vi "read_ini_file.vi"() -> ()   [LabVIEW 2021]
uses:
  <vilib>/Utility/config.llb/Read Key (String).vi
  <vilib>/Utility/config.llb/NI_LVConfig.lvlib
panel:
  out "values":string[][](array[string])
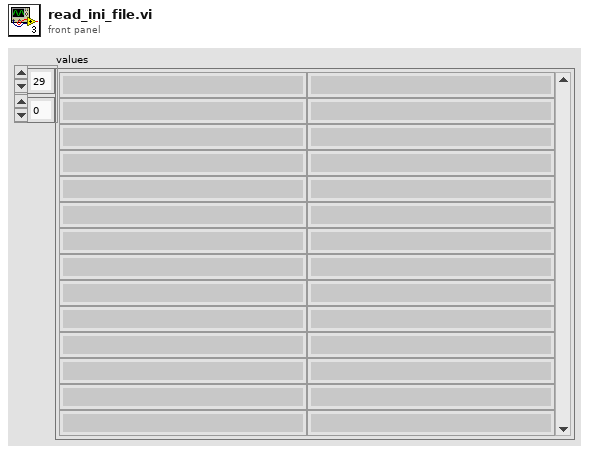
[diagram p1: front panel]
types:
  T1 = typedef "NI_LVConfig.lvlib/Config Data RefNum.ctl" = refnum<k1>
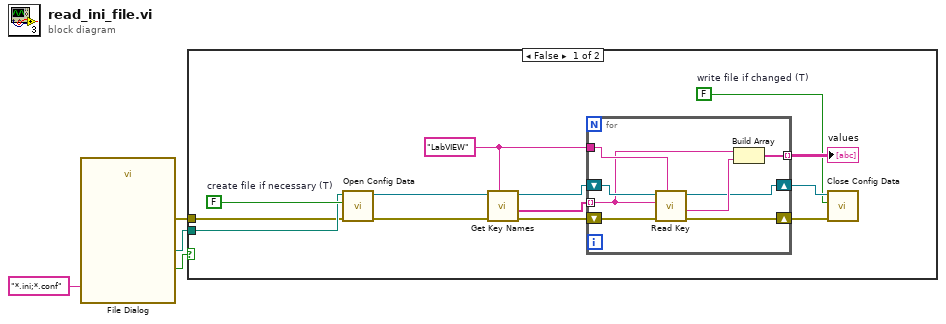
[diagram p0: block diagram]
diagram:
  n1 = call "File Dialog"("pattern (all files)"="*.ini;*.conf") -> ("selected path"=w4:path, "cancelled"=w2:bool, "error out"=w1:errorcluster)  [unwired: 11 in, 1 out]
  n2 = case shown="False" w2 {
    tunnel: w4 -> [w16 _]
    tunnel: w1 -> [w11 _]
    frame False {
      w6 = FALSE  # write file if changed (T)
      w12 = "LabVIEW" ("section")
      w17 = FALSE  # create file if necessary (T)
      n3 = call <vilib>:"Open Config Data.vi"("error in (no error)"=w11, "create file if necessary (T)"=w17, "configuration file path"=w16) -> ("error out"=w10:errorcluster, "refnum"=w14:T1)  [unwired: 6 in, 1 out]
      n4 = call <vilib>:"Get Key Names.vi"("section"=w12, "error in (no error)"=w10, "refnum"=w14) -> ("error out"=w9:errorcluster, "key names"=w15:string[], "refnum out"=w13:T1)  [unwired: 5 in, 1 out]
      n5 = for {
        shift-right: [w21] -> w7
        shift-left: w13 -> [w25]
        tunnel: w15 -> [w23] mode=indexing
        tunnel: w12 -> [w24]
        shift-right: [w19] -> w5
        shift-left: w9 -> [w20]
        tunnel: [w18] -> w8 mode=indexing
        n6 = call-poly <vilib>:"Read Key.vi"("section"=w24, "error in (no error)"=w20, "key"=w23, "refnum"=w25) -> ("error out"=w19:errorcluster, "value"=w22:string, "refnum out"=w21:T1)  [unwired: 4 in, 1 out]
        n7 = Build Array(w23, w22) -> (w18:string[])
      }
      "values" <- w8
      n8 = call <vilib>:"Close Config Data.vi"("error in (no error)"=w5, "write file if changed (T)"=w6, "refnum"=w7) -> ()  [unwired: 7 in, 2 out]
    }
    frame True {
    }
  }
